vi "Vbias Gain Lookup Table.vi"() -> (2 "ROUT<7:5>":u8[](array[numeric])=[7, 6, 5, 4, 0, 1, 2, 3], 3 "VB Gain(dB)":dbl[](array[numeric])=[14.1, 12.6, 13.1, 13.6, 12.1, 11.6, 11.1, 14.1])   [LabVIEW 2020]
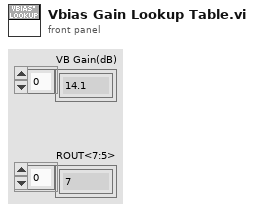
[diagram p1: front panel]
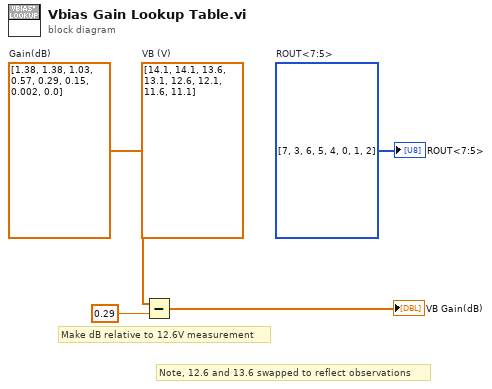
[diagram p0: block diagram]
diagram:
  w3 = dbl[] [1.38, 1.38, 1.03, 0.57, 0.29, 0.15, 0.002, 0.0]  # Gain(dB)
  (unwired) dbl[] [14.1, 14.1, 13.6, 13.1, 12.6, 12.1, 11.6, 11.1]  # VB (V)
  w4 = u8[] [7, 3, 6, 5, 4, 0, 1, 2]  # ROUT<7:5>
  # "Make dB relative to 12.6V measurement"
  # "Note, 12.6 and 13.6 swapped to reflect observations"
  n1 = Subtract(x=w3, y=0.29 ("dB")) -> (x-y=→"VB Gain(dB)":dbl[])
  "ROUT<7:5>" <- w4
